vi "control_622x.vi"() -> ()   [LabVIEW 2018]
uses:
  <instrlib>/Keithley 622x LV 2009/Typedefs/KE622x -- On Off Control.ctl
  <instrlib>/Keithley 622x LV 2009/Keithley 622x.lvlib
panel:
  in  "Commande onglets":enum32{"Settings", "delta", "Hardware"}(tab)
  in  "start":bool
  in  "offset /A":dbl min=-0.1 max=0.1 format="%#.9g"
  in  "Source analog filter":bool
  in  "DMM range /V":dbl=1.0 min=0.01 max=100.0 format="%#.9g"
  in  "compliance /V":dbl=1.0 min=0.1 max=62.0 format="%#.9g"
  in  "AC frequency /Hz":dbl=17.0 min=1e-05 max=100000.0 format="%#.9g"
  in  "current /A (peak)":dbl=1e-09 min=-0.105 max=0.105 format="%#.9g"
  in  "Source autorange":bool
  in  "MODE":enum32{"source DC", "source AC ", "delta "}(radio)
  in  "source":bool
  in  "compliance abort":bool
  in  "DMM autorange":bool
  in  "exit":bool
  out "Graphe":dbl(graph)
  in  "VISA GPIB Resource":refnum<visa-resource-name>="GPIB0::4::INSTR"
  # "frequency TTL output at 0° on line 1\nfor Halbach, use the Trigger 1 connection to the Zurich instruments lock in"
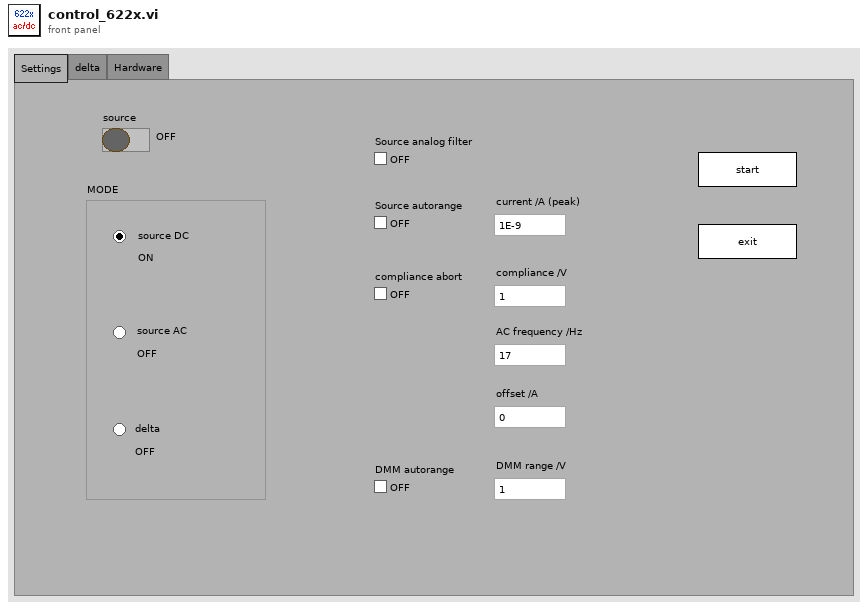
[diagram p1: front panel]
types:
  T1 = enum32{"invalid app kind", "Development System", "Run Time System", "Student Edition", "Embedded LabVIEW", "Evaluation", "Custom"}
  T2 = enum32{"Invalid", "Standard", "Closed", "Hidden", "Minimized", "Maximized"}
  T3 = typedef "Keithley 622x.lvlib/KE622x -- On Off Control.ctl" = enum16{"Off", "On"}
  T4 = cluster{"Core":cluster{"Current VI Reference":refnum<vi>, "Close Panel on Exit?":bool}, "VISA GPIB Resource":refnum<visa-resource-name>, "MODE":enum32{"source DC", "source AC ", "delta "}, "source ":bool, "Source analog filter":bool, "Source autorange ":bool, "compliance abort":bool, "DMM autorange":bool, "current /A (peak)":dbl, "compliance /V":dbl, "AC frequency /Hz":dbl, "DMM range /V ":dbl, "offset /A":dbl, "delta mode ON?":bool}
  T5 = cluster{"Current VI Reference":refnum<vi>, "Close Panel on Exit?":bool}
  T6 = typedef "Keithley 622x.lvlib/KE622x -- Current Range.ctl" = cluster{"Auto Range?":bool, "Man / Selected\nRange":T7}
  T7 = typedef "Keithley 622x.lvlib/KE622x -- Current Ranges.ctl" = enum16{"2nA", "20nA", "200nA", "2uA", "20uA", "200uA", "2mA", "20mA", "100mA"}
  T8 = cluster{"Source autorange ":bool, "Man / Selected\nRange":T7}
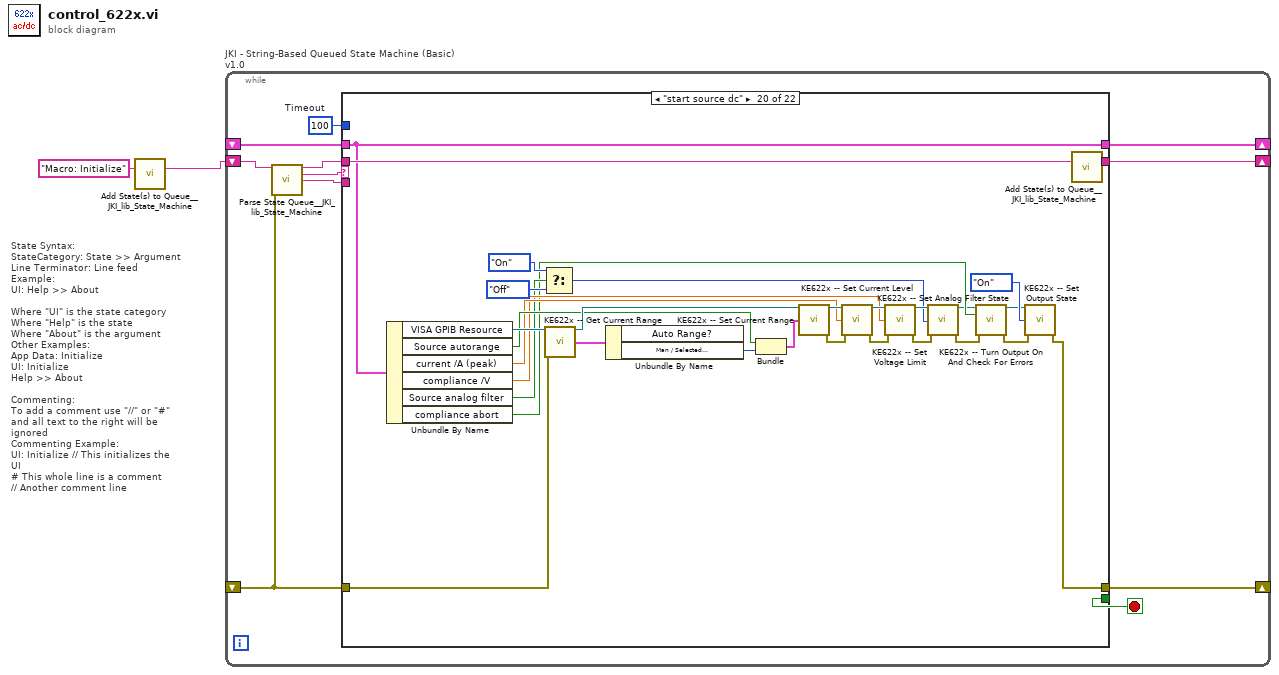
[diagram p0: block diagram]
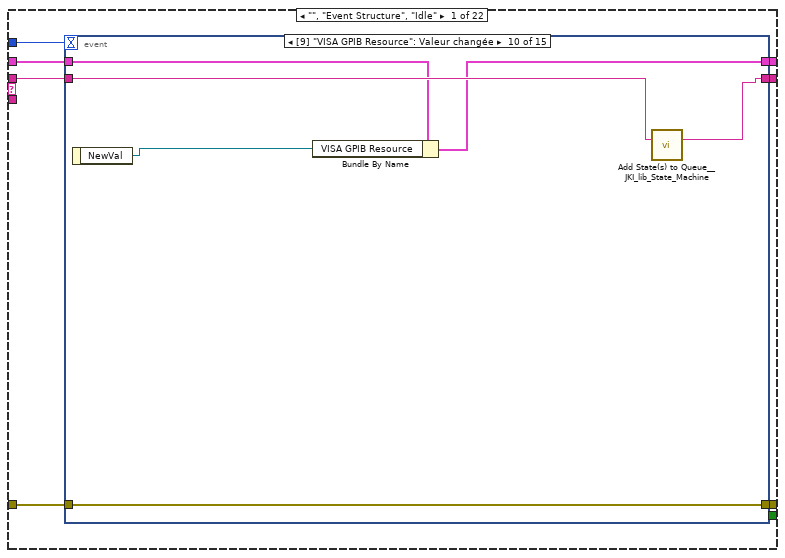
[diagram p2: hidden frame]
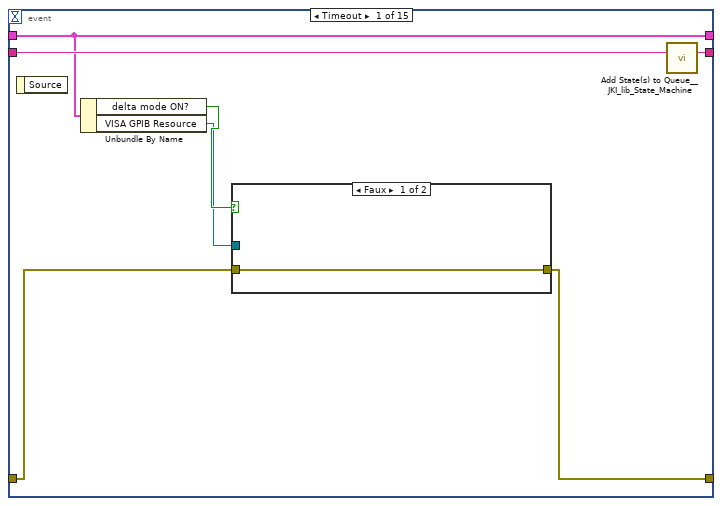
[diagram p3: hidden frame]
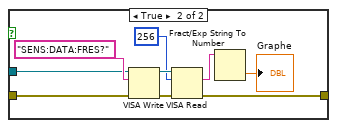
[diagram p4: hidden frame]
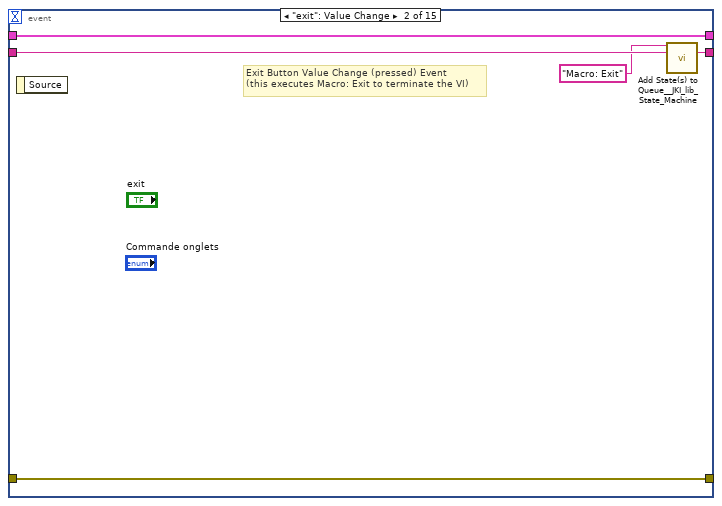
[diagram p5: hidden frame]
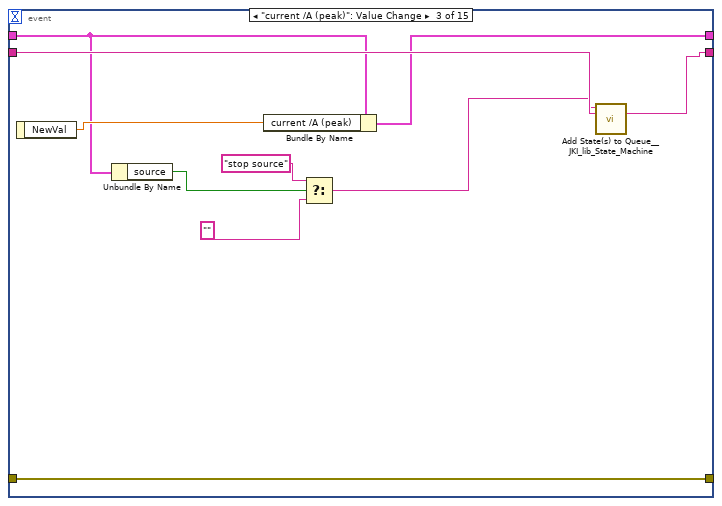
[diagram p6: hidden frame]
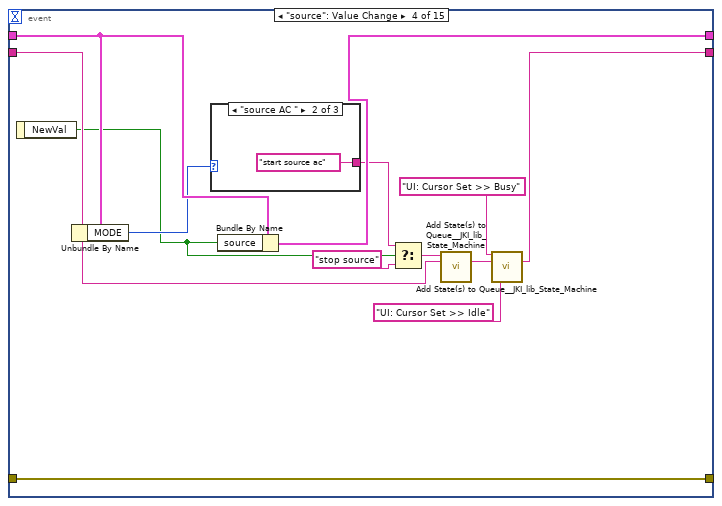
[diagram p7: hidden frame]
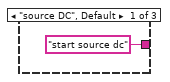
[diagram p8: hidden frame]
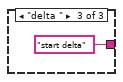
[diagram p9: hidden frame]
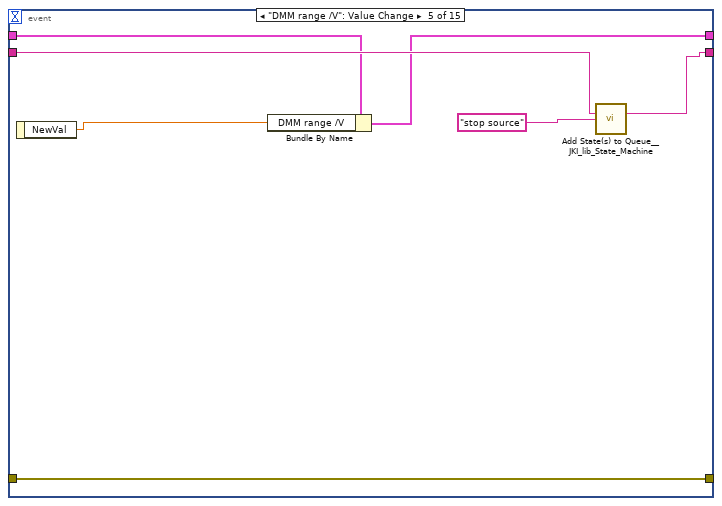
[diagram p10: hidden frame]
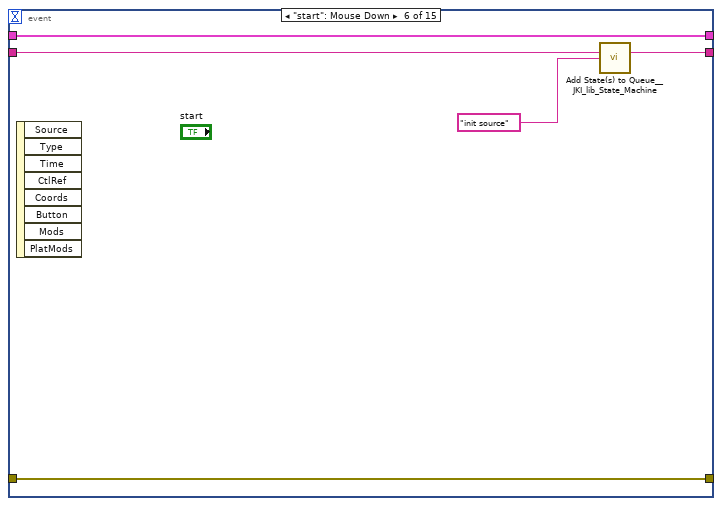
[diagram p11: hidden frame]
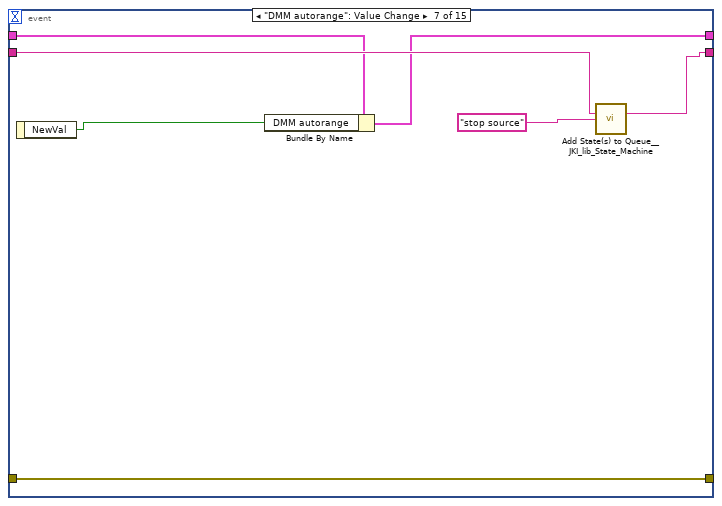
[diagram p12: hidden frame]
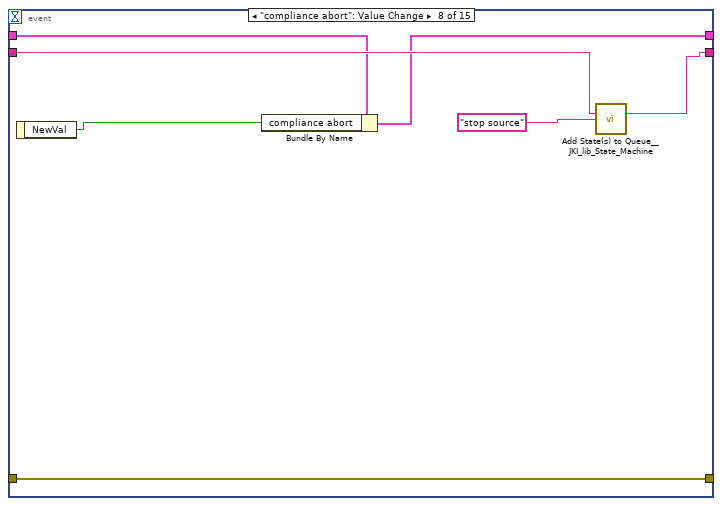
[diagram p13: hidden frame]
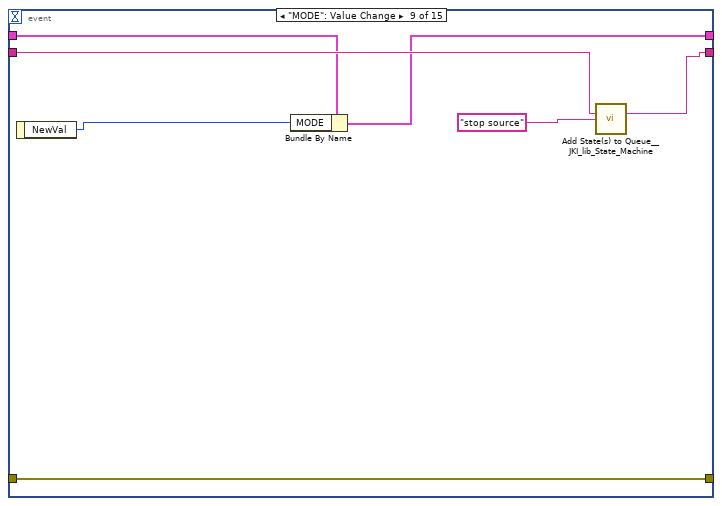
[diagram p14: hidden frame]
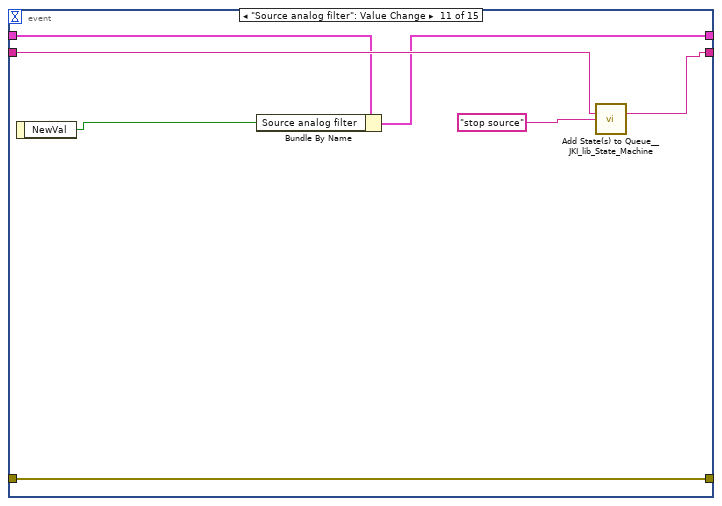
[diagram p15: hidden frame]
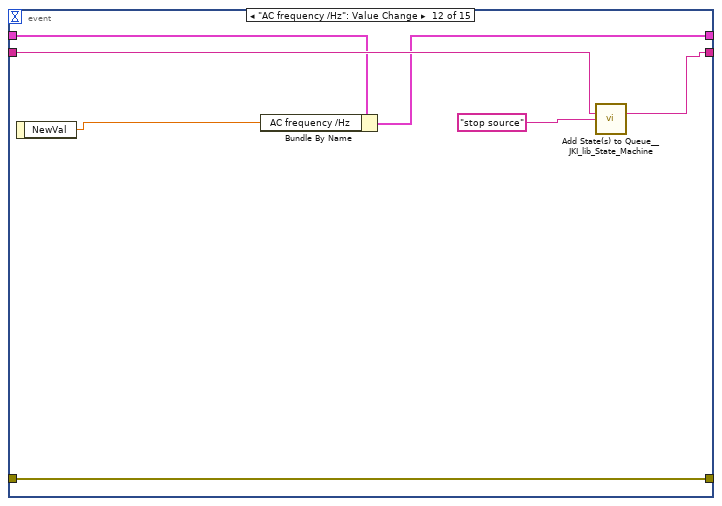
[diagram p16: hidden frame]
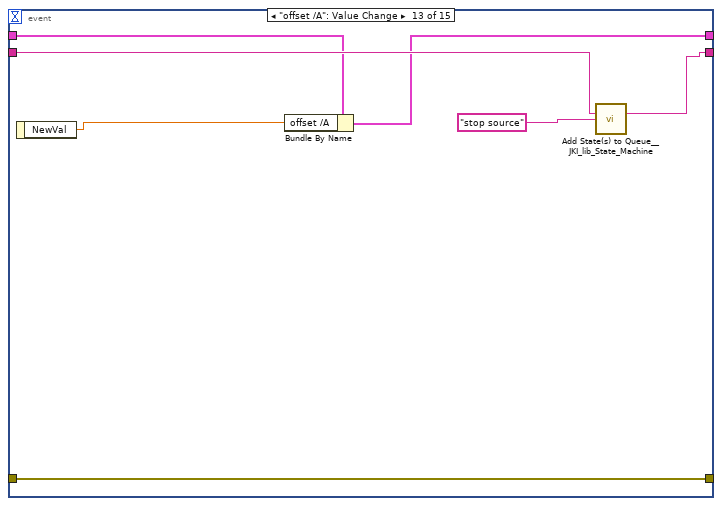
[diagram p17: hidden frame]
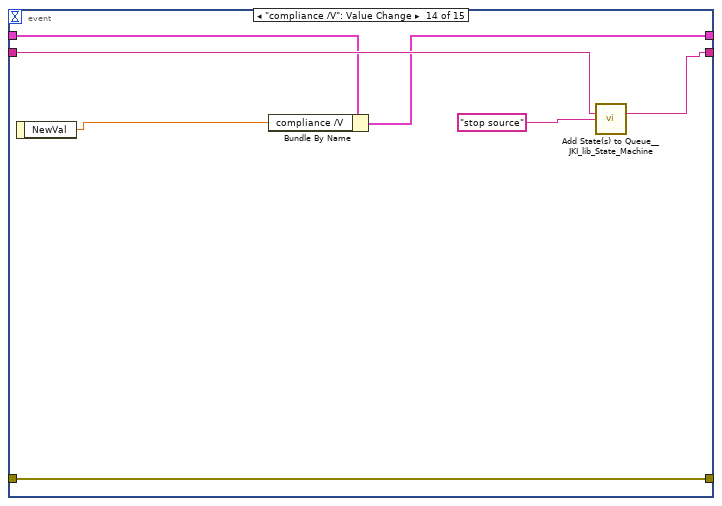
[diagram p18: hidden frame]
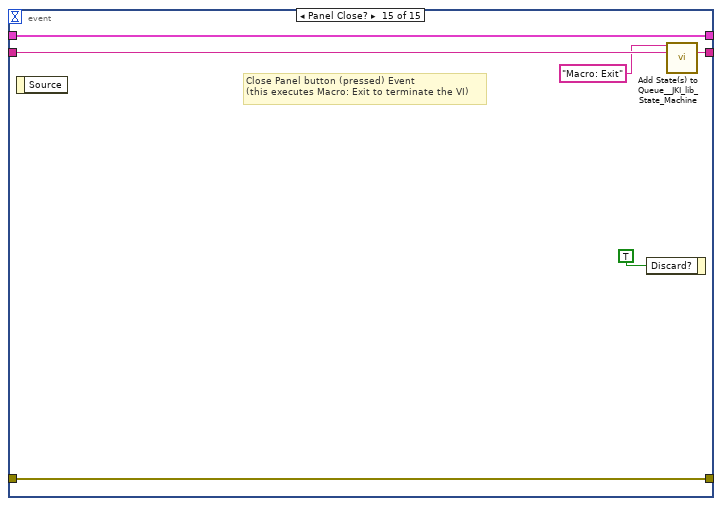
[diagram p19: hidden frame]
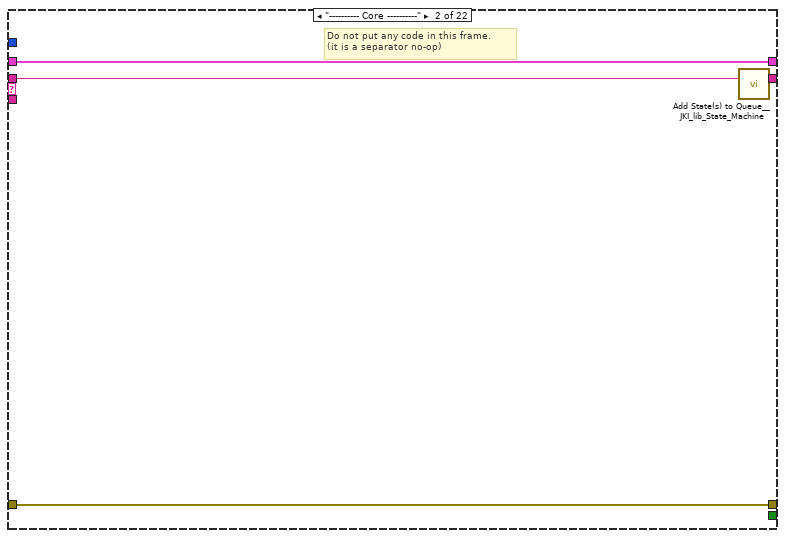
[diagram p20: hidden frame]
diagram:
  # "State Syntax:\nStateCategory: State >> Argument\nLine Terminator: Line feed\nExample:\nUI: Help >> About\n\nWhere \"UI\" is the state category\nWhere \"Help\" is the state\nWhere \"About\" is the argument\nOther Examples:\nApp Data: Initialize\nUI: Initialize\nHelp >> About\n\nCommenting:\nTo add a comment use \"//\" or \"#\" and all text to the right will be ignored\nCommenting Example:\nUI: Initialize // This initializes the UI\n# This whole line is a comment\n// Another comment line"
  n1 = call <vilib>:"Add State(s) to Queue__JKI_lib_State_Machine.vi"("State(s) in (\"\")"="Macro: Initialize") -> ("States Out"=w2:string)  [unwired: 14 in]
  n2 = while "JKI - String-Based Queued State Machine (Basic) v1.0" {
    shift-right: [w7] -> _
    shift-left: _ -> [w6]
    shift-right: [w3] -> _
    shift-left: _ -> [w4]
    shift-right: [w9] -> _
    shift-left: w2 -> [w10]
    stop <- w8 stop-if-true
    w5 = 100  # Timeout
    n3 = call <vilib>:"Parse State Queue__JKI_lib_State_Machine.vi"("State Queue"=w10, "Error In (no error)"=w4) -> ("Remaining States"=w12:string, "Current State"=w13:string, "Arguments"=w11:string)  [unwired: 11 in]
    n4 = case shown="\"start source dc\"" w13 {
      selector: w13 -> [_ _ w146 _ _ _ _ _ _ _ _ _ _ _ _ _ _ _ _ _ _ _]
      tunnel: w12 -> [w20 w145 w150 w168 w174 w179 w183 w201 w207 w211 w215 w221 w232 w258 w263 w274 w278 w291 w310 w339 w349 w362]
      tunnel: w11 -> [_ _ _ _ _ _ _ _ _ _ _ w216 w226 _ _ _ _ _ _ _ _ _]
      tunnel: w6 -> [w18 w142 w148 w159 w171 w177 w180 _ w202 w208 w213 w219 w228 w255 w260 w271 w275 w284 w308 w337 w347 w351]
      tunnel: [w17 w143 w152 w165 errorcluster {"status"=FALSE, "code"=0, "source"=""} ("error out") w176 w181 w184 w203 w209 w212 w217 w229 w256 w261 w272 w276 w280 w299 w311 w340 w355] -> w3
      tunnel: w4 -> [w16 w143 w151 w165 w170 w176 w181 w184 w204 w209 w212 w218 w230 w256 w261 w272 w276 w285 w301 w312 w341 w356]
      tunnel: [w19 w144 w149 w167 w173 w178 w182 w200 w206 w210 w214 w220 w231 w257 w262 w273 w277 w290 w309 w338 w348 w361] -> w9
      tunnel: [_ _ _ _ _ TRUE _ _ _ _ _ _ _ _ _ _ _ _ _ _ _ _] -> w8
      tunnel: [w15 w142 w148 w166 w171 w177 w180 w199 w202 w208 w213 w219 w228 w255 w260 w271 w275 w283 w308 w337 w347 w350] -> w7
      tunnel: w5 -> [w14 _ _ _ _ _ _ _ _ _ _ _ _ _ _ _ _ _ _ _ _ _]
      frame "", "Event Structure", "Idle" {
        n5 = event shown="[9] \"VISA GPIB Resource\": Valeur changée" {
          selector: _ -> [_ _ _ _ _ _ _ _ _ _ _ _ _ _ _]
          dyn-events: _ -> [_ _ _ _ _ _ _ _ _ _ _ _ _ _ _]
          timeout: w14 -> [_ _ _ _ _ _ _ _ _ _ _ _ _ _ _]
          tunnel: w20 -> [w27 w42 w51 w65 w73 w78 w85 w92 w99 w106 w112 w119 w126 w133 w141]
          tunnel: [w26 w41 w52 w57 w75 w80 w87 w94 w101 w107 w114 w121 w128 w135 w140] -> w19
          tunnel: w18 -> [w25 w39 w47 w62 w72 w76 w84 w91 w98 w105 w111 w118 w125 w132 w138]
          tunnel: [w21 w40 w48 w63 w69 w77 w81 w88 w95 w102 w108 w115 w122 w129 w139] -> w17
          tunnel: w16 -> [w22 w40 w48 w63 w69 w77 w81 w88 w95 w102 w108 w115 w122 w129 w139]
          tunnel: [w25 w39 w50 w64 w71 w76 w83 w90 w97 w104 w110 w117 w124 w131 w138] -> w15
          event Timeout {
            n6 = event-data() -> ()  [unwired: 1 in, 1 out]
            n7 = Unbundle By Name(w25) -> ("delta mode ON?"=w24:bool, "VISA GPIB Resource"=w23:refnum<visa-resource-name>)
            n8 = case shown="Faux" w24 {
              tunnel: w23 -> [_ w32]
              tunnel: w22 -> [w28 w31]
              tunnel: [w28 w30] -> w21
              frame False {
              }
              frame True {
                n9 = VISA Write(VISA resource name=w32, write buffer="SENS:DATA:FRES?" ("buffer d'écriture"), error in (no error)=w31) -> (VISA resource name out=w36:refnum<visa-resource-name>, error out=w35:errorcluster)  [unwired: 1 out]
                n10 = VISA Read(VISA resource name=w36, byte count=u32 256 ("nombre d'octets"), error in (no error)=w35) -> (read buffer=w33:string, error out=w30:errorcluster)  [unwired: 2 out]
                n11 = Fract/Exp String To Number(string=w33) -> (number=→"Graphe":dbl)  [unwired: 3 in, 1 out]
              }
            }
            n12 = call <vilib>:"Add State(s) to Queue__JKI_lib_State_Machine.vi"("State(s) in (\"\")"=w27) -> ("States Out"=w26:string)  [unwired: 14 in]
          }
          event "exit": Value Change {
            # "Exit Button Value Change (pressed) Event\n(this executes Macro: Exit to terminate the VI)"
            n13 = event-data() -> ()  [unwired: 1 in, 1 out]
            n14 = call <vilib>:"Add State(s) to Queue__JKI_lib_State_Machine.vi"("State(s) in Front (\"\")"="Macro: Exit", "State(s) in (\"\")"=w42) -> ("States Out"=w41:string)  [unwired: 13 in]
          }
          event "current /A (peak)": Value Change {
            n15 = event-data() -> ("NewVal"=w49:dbl)  [unwired: 1 in]
            n16 = Unbundle By Name(w47) -> ("source"=w46:bool)
            n17 = Bundle By Name(cluster=w47, "current /A (peak)"=w49) -> (w50:T4)
            n18 = Select(t="stop source", s=w46, f="") -> (s? t:f=w43:string)
            n19 = call <vilib>:"Add State(s) to Queue__JKI_lib_State_Machine.vi"("State(s) in Front (\"\")"=w43, "State(s) in (\"\")"=w51) -> ("States Out"=w52:string)  [unwired: 13 in]
          }
          event "source": Value Change {
            n20 = event-data() -> ("NewVal"=w53:bool)  [unwired: 1 in]
            n21 = Unbundle By Name(w62) -> ("MODE"=w59:enum32{"source DC", "source AC ", "delta "})
            n22 = case shown="\"source AC \"" w59 {
              tunnel: ["start source dc" "start source ac" "start delta"] -> w58
              frame "source DC", Default {
              }
              frame "source AC " {
              }
              frame "delta " {
              }
            }
            n23 = Bundle By Name(cluster=w62, "source"=w53) -> (w64:T4)
            n24 = Select(t=w58, s=w53, f="stop source") -> (s? t:f=w61:string)
            n25 = call <vilib>:"Add State(s) to Queue__JKI_lib_State_Machine.vi"("State(s) in Front (\"\")"=w61, "State(s) in (\"\")"=w65) -> ("States Out"=w56:string)  [unwired: 13 in]
            n26 = call <vilib>:"Add State(s) to Queue__JKI_lib_State_Machine.vi"("State(s) in Front (\"\")"="UI: Cursor Set >> Busy", "State(s) in (\"\")"=w56, "State(s) at Back (\"\")"="UI: Cursor Set >> Idle") -> ("States Out"=w57:string)  [unwired: 12 in]
          }
          event "DMM range /V": Value Change {
            n27 = event-data() -> ("NewVal"=w70:dbl)  [unwired: 1 in]
            n28 = Bundle By Name(cluster=w72, "DMM range /V"=w70) -> (w71:T4)
            n29 = call <vilib>:"Add State(s) to Queue__JKI_lib_State_Machine.vi"("State(s) in (\"\")"=w73, "State(s) at Back (\"\")"="stop source") -> ("States Out"=w75:string)  [unwired: 13 in]
          }
          event "start": Mouse Down {
            n30 = event-data() -> ()  [unwired: 1 in, 8 out]
            n31 = call <vilib>:"Add State(s) to Queue__JKI_lib_State_Machine.vi"("State(s) in (\"\")"=w78, "State(s) at Back (\"\")"="init source") -> ("States Out"=w80:string)  [unwired: 13 in]
          }
          event "DMM autorange": Value Change {
            n32 = event-data() -> ("NewVal"=w82:bool)  [unwired: 1 in]
            n33 = Bundle By Name(cluster=w84, "DMM autorange"=w82) -> (w83:T4)
            n34 = call <vilib>:"Add State(s) to Queue__JKI_lib_State_Machine.vi"("State(s) in (\"\")"=w85, "State(s) at Back (\"\")"="stop source") -> ("States Out"=w87:string)  [unwired: 13 in]
          }
          event "compliance abort": Value Change {
            n35 = event-data() -> ("NewVal"=w89:bool)  [unwired: 1 in]
            n36 = Bundle By Name(cluster=w91, "compliance abort"=w89) -> (w90:T4)
            n37 = call <vilib>:"Add State(s) to Queue__JKI_lib_State_Machine.vi"("State(s) in (\"\")"=w92, "State(s) at Back (\"\")"="stop source") -> ("States Out"=w94:string)  [unwired: 13 in]
          }
          event "MODE": Value Change {
            n38 = event-data() -> ("NewVal"=w96:enum32{"source DC", "source AC ", "delta "})  [unwired: 1 in]
            n39 = Bundle By Name(cluster=w98, "MODE"=w96) -> (w97:T4)
            n40 = call <vilib>:"Add State(s) to Queue__JKI_lib_State_Machine.vi"("State(s) in (\"\")"=w99, "State(s) at Back (\"\")"="stop source") -> ("States Out"=w101:string)  [unwired: 13 in]
          }
          event "VISA GPIB Resource": Value Change {
            n41 = event-data() -> ("NewVal"=w103:refnum<visa-resource-name>)  [unwired: 1 in]
            n42 = Bundle By Name(cluster=w105, "VISA GPIB Resource"=w103) -> (w104:T4)
            n43 = call <vilib>:"Add State(s) to Queue__JKI_lib_State_Machine.vi"("State(s) in (\"\")"=w106) -> ("States Out"=w107:string)  [unwired: 14 in]
          }
          event "Source analog filter": Value Change {
            n44 = event-data() -> ("NewVal"=w109:bool)  [unwired: 1 in]
            n45 = Bundle By Name(cluster=w111, "Source analog filter"=w109) -> (w110:T4)
            n46 = call <vilib>:"Add State(s) to Queue__JKI_lib_State_Machine.vi"("State(s) in (\"\")"=w112, "State(s) at Back (\"\")"="stop source") -> ("States Out"=w114:string)  [unwired: 13 in]
          }
          event "AC frequency /Hz": Value Change {
            n47 = event-data() -> ("NewVal"=w116:dbl)  [unwired: 1 in]
            n48 = Bundle By Name(cluster=w118, "AC frequency /Hz"=w116) -> (w117:T4)
            n49 = call <vilib>:"Add State(s) to Queue__JKI_lib_State_Machine.vi"("State(s) in (\"\")"=w119, "State(s) at Back (\"\")"="stop source") -> ("States Out"=w121:string)  [unwired: 13 in]
          }
          event "offset /A": Value Change {
            n50 = event-data() -> ("NewVal"=w123:dbl)  [unwired: 1 in]
            n51 = Bundle By Name(cluster=w125, "offset /A"=w123) -> (w124:T4)
            n52 = call <vilib>:"Add State(s) to Queue__JKI_lib_State_Machine.vi"("State(s) in (\"\")"=w126, "State(s) at Back (\"\")"="stop source") -> ("States Out"=w128:string)  [unwired: 13 in]
          }
          event "compliance /V": Value Change {
            n53 = event-data() -> ("NewVal"=w130:dbl)  [unwired: 1 in]
            n54 = Bundle By Name(cluster=w132, "compliance /V"=w130) -> (w131:T4)
            n55 = call <vilib>:"Add State(s) to Queue__JKI_lib_State_Machine.vi"("State(s) in (\"\")"=w133, "State(s) at Back (\"\")"="stop source") -> ("States Out"=w135:string)  [unwired: 13 in]
          }
          event Panel Close? {
            # "Close Panel button (pressed) Event\n(this executes Macro: Exit to terminate the VI)"
            n56 = event-data() -> ()  [unwired: 1 in, 1 out]
            n57 = event-data("Discard?"=TRUE) -> ()  [unwired: 1 in, 1 out]
            n58 = call <vilib>:"Add State(s) to Queue__JKI_lib_State_Machine.vi"("State(s) in Front (\"\")"="Macro: Exit", "State(s) in (\"\")"=w141) -> ("States Out"=w140:string)  [unwired: 13 in]
          }
        }
      }
      frame "---------- Core ----------" {
        # "Do not put any code in this frame.\n(it is a separator no-op)"
        n59 = call <vilib>:"Add State(s) to Queue__JKI_lib_State_Machine.vi"("State(s) in (\"\")"=w145) -> ("States Out"=w144:string)  [unwired: 14 in]
      }
      frame Default {
        w155 = 42 items=["No error", "Argument error", "Memory is full", "Out of zone", "End of file", "File already open", "Generic file I/O error", "File not found", "File permission error", "Disk is full", "Duplicate path", "Too many files open", "System feature not enabled", "Resource file not found", "Cannot add resource", "Resource not found", "Image not found", "Image memory error", "Pen does not exist", "Config type invalid", "Config token not found", "Config parse error", "Config memory error", "Bad external code format", "Bad external code offset", "External code not present", "Null window", "Destroy window error", "Null menu", "Print aborted", "Bad print record", "Print driver error", "Windows error during printing", "Memory error during printing", "Print dialog error", "Generic print error", "Invalid device refnum", "Device not found", "Device parameter error", "Device unit error", "Cannot open device", "Device call aborted", "Generic error", "Cancelled by user", "Object ID too low", "Object ID too high", "Object not in heap", "Unknown heap", "Unknown object (invalid DefProc)", "Unknown object (DefProc not in table)", "Message out of range", "Invalid (null) method", "Unknown message", "Manager call not supported", "Bad address", "Network operation in progress", "Network operation timed out", "Connection is busy", "Network attribute not supported", "Network error", "Address in use", "System out of memory", "Connection aborted", "Connection refused", "Not connected", "Already connected", "Connection closed", "Initialization error (interapplication manager)", "Bad occurrence", "Wait on unbound occurrence handler", "Occurrence queue overflow", "Datalog type conflict", "Unused", "Unrecognized type (interapplication manager)", "Memory corrupt", "Failed to make temporary DLL", "Old CIN version", "Drag socket not found", "Failed to load drop-object", "Failed to register OLE object", "Failed to release OLE object", "Format specifier type mismatch", "Unknown format specifier", "Too few format specifiers", "Too many format specifiers", "Scan failed", "Newer CIN version", "Error converting to variant", "Runtime menu error", "Password tampered", "Variant attribute not found", "Incompatible variant data type", "Event data is not available", "Event Store is not present", "Occurrence is not found", "Event Queue is not created", "Event info is not available", "Refnum passed is NULL", "Error retrieving Class GUID", "Error retrieving CoClass GUID", "Error retrieving TypeLib GUID.", "Bad built application magic bytes.", "Specific driver is different from the specific driver associated with the Logical Name.", "There is no session opened to the class driver.", "Max Error", "MAX - Error with config objects", "MAX - Error loading configuration", "MAX - Group not supported"]
        # "Current State"
        # "Do not delete, rename, or modify this frame.\n(this is used to capture unhandled states and typos)"
        # "Handle mistyped state name (developer tool)"
        n60 = Format Into String(format string="Software Exception: Unhandled State \"%s\"." ("message"), error in=w151, w146) -> (resulting string=w154:string, error out=w153:errorcluster)  [unwired: 1 in]
        n61 = call <vilib>:"Error Cluster From Error Code.vi"("show call chain? (False)"=TRUE, "error in (no error)"=w153, "error message (\"\")"=w154, "error code (0)"=w155) -> ("error out"=w152:errorcluster)  [unwired: 5 in]
        n62 = call <vilib>:"Add State(s) to Queue__JKI_lib_State_Machine.vi"("State(s) in (\"\")"=w150) -> ("States Out"=w149:string)  [unwired: 14 in]
      }
      frame "Initialize Core Data" {
        # "Do not delete, rename, or modify this frame.\n(this is used to determine panel behavior on exit)"
        # "originally closed?"
        # "exe?"
        # "If panel starts closed or is an EXE, then close it when we exit"
        n63 = property class="VI"() -> ("Front Panel.Open"=w164:bool)  [unwired: 2 in, 2 out]
        n64 = property class="App"() -> ("App.Kind"=w163:T1)  [unwired: 2 in, 2 out]
        n65 = control-ref of="Current VI Reference"() -> (w157:refnum<vi>)
        n66 = Not(x=w164) -> (.not. x?=w161:bool)
        n67 = Equal?(x=w163, y=T1."Run Time System" ("Application:Kind")) -> (x = y?=w160:bool)
        n68 = Or(x=w161, y=w160) -> (x .or. y?=w158:bool)
        n69 = Bundle By Name(cluster=w159, "Core.Current VI Reference"=w157, "Core.Close Panel on Exit?"=w158) -> (w166:T4)
        n70 = call <vilib>:"Add State(s) to Queue__JKI_lib_State_Machine.vi"("State(s) in (\"\")"=w168) -> ("States Out"=w167:string)  [unwired: 14 in]
      }
      frame "Error Handler" {
        # "Unhandled Error -- Display it"
        # "Handle any errors here.\nYou can also output any states to clean-up after errors occur"
        # "Clear error"
        n71 = call <vilib>:"General Error Handler.vi"("error in (no error)"=w170) -> ()  [unwired: 10 in, 5 out]
        n72 = call <vilib>:"Add State(s) to Queue__JKI_lib_State_Machine.vi"("State(s) in Front (\"\")"="/* Post Error States", "State(s) in (\"\")"=w174) -> ("States Out"=w173:string)  [unwired: 13 in]
      }
      frame "Exit" {
        # "Do not put any code in this frame.\n(No errors that occur here will be handled.)"
        n73 = call <vilib>:"Add State(s) to Queue__JKI_lib_State_Machine.vi"("State(s) in (\"\")"=w179) -> ("States Out"=w178:string)  [unwired: 14 in]
      }
      frame "---------- Data ----------" {
        # "Do not put any code in this frame.\n(It is a separator no-op. You can make a copy of this frame to create a new Data frame)"
        n74 = call <vilib>:"Add State(s) to Queue__JKI_lib_State_Machine.vi"("State(s) in (\"\")"=w183) -> ("States Out"=w182:string)  [unwired: 14 in]
      }
      frame "Data: Initialize" {
        w185 = FALSE  # delta mode ON?
        w198 = T5 {"Current VI Reference"=refnum, "Close Panel on Exit?"=FALSE}  # Core
        # "Initialize the shift-register data, here.\n(data names are defined by what you wire into the bundle function)"
        n75 = Bundle("Core"=w198, "VISA GPIB Resource"="VISA GPIB Resource", "MODE"="MODE", "source"="source", "Source analog filter"="Source analog filter", "Source autorange"="Source autorange", "compliance abort"="compliance abort", "DMM autorange"="DMM autorange", "current /A (peak)"="current /A (peak)", "compliance /V"="compliance /V", "AC frequency /Hz"="AC frequency /Hz", "DMM range /V"="DMM range /V", "offset /A"="offset /A", "delta mode ON?"=w185) -> (w199:T4)  [unwired: 1 in]
        n76 = call <vilib>:"Add State(s) to Queue__JKI_lib_State_Machine.vi"("State(s) in (\"\")"=w201) -> ("States Out"=w200:string)  [unwired: 14 in]
      }
      frame "Data: Cleanup" {
        # "Cleanup any data and references, here.\n(this is called automatically, by the Macro: Exit)"
        n77 = Unbundle By Name(w202) -> ("Core.Current VI Reference"=w205:refnum<vi>)
        n78 = Close Reference(reference=w205, error in (no error)=w204) -> (error out=w203:errorcluster)
        n79 = call <vilib>:"Add State(s) to Queue__JKI_lib_State_Machine.vi"("State(s) in (\"\")"=w207) -> ("States Out"=w206:string)  [unwired: 14 in]
      }
      frame "---------- UI ----------" {
        # "Do not put any code in this frame.\n(It is a separator no-op. You can make a copy of this frame to create a new UI frame)"
        n80 = call <vilib>:"Add State(s) to Queue__JKI_lib_State_Machine.vi"("State(s) in (\"\")"=w211) -> ("States Out"=w210:string)  [unwired: 14 in]
      }
      frame "UI: Initialize" {
        # "Initialize the User Interface, here.\n(this is called automatically, by the Macro: Init)"
        n81 = call <vilib>:"Add State(s) to Queue__JKI_lib_State_Machine.vi"("State(s) in (\"\")"=w215) -> ("States Out"=w214:string)  [unwired: 14 in]
      }
      frame "UI: Cursor Set" {
        # "Argument"
        # "Set and Unset Cursor Busy.\n(Usage: \"UI: Cursor Set >> Busy|Idle\")"
        n82 = case shown="\"Idle\", Par défaut" w216 {
          tunnel: w218 -> [w223 w225]
          tunnel: [w222 w224] -> w217
          frame "Idle", Default {
            n83 = call <vilib>:"Unset Busy.vi"("error in (no error)"=w223) -> ("error out"=w222:errorcluster)  [unwired: 10 in]
          }
          frame "Busy" {
            n84 = call <vilib>:"Set Busy.vi"("error in (no error)"=w225) -> ("error out"=w224:errorcluster)  [unwired: 9 in, 1 out]
          }
        }
        n85 = call <vilib>:"Add State(s) to Queue__JKI_lib_State_Machine.vi"("State(s) in (\"\")"=w221) -> ("States Out"=w220:string)  [unwired: 14 in]
      }
      frame "UI: Front Panel State" {
        # "Argument"
        # "Set Front Panel Open or Closed\n(Usage: \"UI: Front Panel State >> Open|Close\")"
        n86 = Unbundle By Name(w228) -> ("Core.Current VI Reference"=w227:refnum<vi>)
        n87 = case shown="\"Open\", Par défaut" w226 {
          tunnel: w230 -> [w236 w249]
          tunnel: [w238 w250] -> w229
          tunnel: w227 -> [w237 w247]
          frame "Open", Default {
            n88 = property class="VI"(reference=w237, error in=w236) -> (reference out=w234:refnum<vi>, error out=w235:errorcluster, "Front Panel.Open"=w233:bool)
            n89 = case shown="Vrai" w233 {
              tunnel: [w241 w244] -> w238
              tunnel: w235 -> [w240 w244]
              tunnel: w234 -> [w239 _]
              frame False {
                n90 = invoke class="VI" method="FA.Ouvrir"(reference=w239, error in=w240, "Activate"=TRUE, "State"=T2."Standard") -> (error out=w241:errorcluster)  [unwired: 1 in, 4 out]
              }
              frame True {
              }
            }
          }
          frame "Close" {
            n91 = property class="VI"(reference=w247, error in=w249) -> (reference out=w246:refnum<vi>, error out=w248:errorcluster, "Front Panel.Open"=w245:bool)
            n92 = case shown="Vrai" w245 {
              tunnel: [w251 w254] -> w250
              tunnel: w248 -> [w251 w253]
              tunnel: w246 -> [_ w252]
              frame False {
              }
              frame True {
                n93 = invoke class="VI" method="FA.Fermer"(reference=w252, error in=w253) -> (error out=w254:errorcluster)  [unwired: 1 in, 2 out]
              }
            }
          }
        }
        n94 = call <vilib>:"Add State(s) to Queue__JKI_lib_State_Machine.vi"("State(s) in (\"\")"=w232) -> ("States Out"=w231:string)  [unwired: 14 in]
      }
      frame "---------- Macro ----------" {
        # "Do not put any code in this frame.\n(It is a separator no-op. You can make a copy of this frame to create a new Macro frame)"
        n95 = call <vilib>:"Add State(s) to Queue__JKI_lib_State_Machine.vi"("State(s) in (\"\")"=w258) -> ("States Out"=w257:string)  [unwired: 14 in]
      }
      frame "Macro: Initialize" {
        # "Initialization Macro\n(This is called once, when the VI starts)"
        n96 = call <vilib>:"Add State(s) to Queue__JKI_lib_State_Machine.vi"("State(s) in Front (\"\")"="UI: Cursor Set >> Busy\nData: Initialize\nInitialize Core Data\nUI: Initialize\nUI: Front Panel State >> Open\nUI: Cursor Set >> Idle", "State(s) in (\"\")"=w263) -> ("States Out"=w262:string)  [unwired: 13 in]
      }
      frame "Macro: Exit" {
        # "Exit Macro\n(This is called once, when the VI exits)"
        n97 = Unbundle By Name(w271) -> ("Core.Close Panel on Exit?"=w270:bool)
        n98 = Select(t="UI: Front Panel State >> Close", s=w270, f="") -> (s? t:f=w267:string)
        n99 = call <vilib>:"Add State(s) to Queue__JKI_lib_State_Machine.vi"("State(s) in Front (\"\")"="stop source" ("State(s) in Front (\"\")"), "State(s) in (\"\")"=w267, "State(s) at Back (\"\")"="Data: Cleanup\nExit") -> ("States Out"=w265:string)  [unwired: 12 in]
        n100 = call <vilib>:"Add State(s) to Queue__JKI_lib_State_Machine.vi"("State(s) in Front (\"\")"=w265, "State(s) in (\"\")"=w274) -> ("States Out"=w273:string)  [unwired: 13 in]
      }
      frame "---------- my state machine ----------" {
        # "Template Separator\n(You can make a copy of, or modify, this frame)"
        n101 = call <vilib>:"Add State(s) to Queue__JKI_lib_State_Machine.vi"("State(s) in (\"\")"=w278) -> ("States Out"=w277:string)  [unwired: 14 in]
      }
      frame "stop source" {
        # "clear error if the source is not active"
        n102 = Unbundle By Name(w284) -> ("VISA GPIB Resource"=w289:refnum<visa-resource-name>)
        n103 = call <instrlib>:"KE622x -- Get Output State.vi"("Resource In"=w289, "error in (no error)"=w285) -> ("Resource Out (dupl)"=w287:refnum<visa-resource-name>, "Output State"=w288:T3, "error out"=w286:errorcluster)  [unwired: 11 in]
        n104 = case shown="\"Off\", Par défaut" w288 {
          tunnel: w287 -> [_ w297]
          tunnel: w286 -> [w292 w296]
          tunnel: [w292 w293] -> w281
          frame "Off", Default {
          }
          frame "On" {
            n105 = call <instrlib>:"KE622x -- Set Output State.vi"("Resource In"=w297, "Output State"=KE622x_--_On_Off_Control."Off", "error in (no error)"=w296) -> ("error out"=w294:errorcluster)  [unwired: 11 in, 1 out]
            n106 = property on="source" class="Bool (strict)"(error in=w294, "Value"=FALSE ("source on")) -> (error out=w293:errorcluster)  [unwired: 1 in, 1 out]
          }
        }
        n107 = Bundle By Name(cluster=w284, "delta mode ON?"=FALSE) -> (w283:T4)
        n108 = call <vilib>:"Clear Errors.vi"("error in (no error)"=w281, "specific error code to clear (0: all)"=0) -> ("error out"=w280:errorcluster)  [unwired: 4 in, 1 out]
        n109 = call <vilib>:"Add State(s) to Queue__JKI_lib_State_Machine.vi"("State(s) in (\"\")"=w291) -> ("States Out"=w290:string)  [unwired: 14 in]
      }
      frame "init source" {
        n110 = Unbundle By Name(w308) -> ("VISA GPIB Resource"=w300:refnum<visa-resource-name>)
        n111 = VISA Write(VISA resource name=w300, write buffer=":sour:wave:abor\n:outp:stat off\n*rst" ("buffer à écrire"), error in (no error)=w301) -> (VISA resource name out=w302:refnum<visa-resource-name>, error out=w304:errorcluster)  [unwired: 1 out]
        n112 = call "wait"("error in (no error)"=w304, "Delay Time (s)"=1.0) -> ("error out"=w303:errorcluster)  [unwired: 9 out]
        n113 = VISA Write(VISA resource name=w302, write buffer=":outp:ish olow\n:outp:lte off" ("buffer à écrire"), error in (no error)=w303) -> (error out=w299:errorcluster)  [unwired: 2 out]
        n114 = call <vilib>:"Add State(s) to Queue__JKI_lib_State_Machine.vi"("State(s) in (\"\")"=w310) -> ("States Out"=w309:string)  [unwired: 14 in]
      }
      frame "start source dc" {
        n115 = Unbundle By Name(w337) -> ("VISA GPIB Resource"=w333:refnum<visa-resource-name>, "Source autorange"=w329:bool, "current /A (peak)"=w327:dbl, "compliance /V"=w326:dbl, "Source analog filter"=w323:bool, "compliance abort"=w318:bool)
        n116 = Select(t=KE622x_--_On_Off_Control."On" ("Analog Filter State"), s=w323, f=KE622x_--_On_Off_Control."Off" ("Analog Filter State")) -> (s? t:f=w322:T3)
        n117 = call <instrlib>:"KE622x -- Get Current Range.vi"("Resource In"=w333, "error in (no error)"=w312) -> ("Resource Out (dupl)"=w332:refnum<visa-resource-name>, "Current Range"=w331:T6)  [unwired: 11 in, 1 out]
        n118 = Unbundle By Name(w331) -> ("Man / Selected\nRange"=w330:T7)  [unwired: 1 out]
        n119 = Bundle("Source autorange"=w329, "Man / Selected\nRange"=w330) -> (w328:T8)  [unwired: 1 in]
        n120 = call <instrlib>:"KE622x -- Set Current Range.vi"("Resource In"=w332, "Current Range In"=w328) -> ("Resource Out (dupl)"=w336:refnum<visa-resource-name>, "error out"=w320:errorcluster)  [unwired: 11 in, 1 out]
        n121 = call <instrlib>:"KE622x -- Set Current Level.vi"("Resource In"=w336, "Current Level (A) In"=w327, "error in (no error)"=w320) -> ("Resource Out (dupl)"=w335:refnum<visa-resource-name>, "error out"=w319:errorcluster)  [unwired: 10 in, 1 out]
        n122 = call <instrlib>:"KE622x -- Set Voltage Limit.vi"("Resource In"=w335, "Voltage Limit (V)"=w326, "error in (no error)"=w319) -> ("Resource Out (dupl)"=w334:refnum<visa-resource-name>, "error out"=w315:errorcluster)  [unwired: 11 in]
        n123 = call <instrlib>:"KE622x -- Set Analog Filter State.vi"("Resource In"=w334, "Analog Filter State"=w322, "error in (no error)"=w315) -> ("Resource Out (dupl)"=w317:refnum<visa-resource-name>, "error out"=w314:errorcluster)  [unwired: 11 in]
        n124 = call <instrlib>:"KE622x -- Turn Output On And Check For Errors.vi"("Resource In"=w317, "Turn Off Output If Compliance?"=w318, "error in (no error)"=w314) -> ("Resource Out (dupl)"=w316:refnum<visa-resource-name>, "error out"=w313:errorcluster)  [unwired: 9 in, 2 out]
        n125 = call <instrlib>:"KE622x -- Set Output State.vi"("Resource In"=w316, "Output State"=KE622x_--_On_Off_Control."On", "error in (no error)"=w313) -> ("error out"=w311:errorcluster)  [unwired: 11 in, 1 out]
        n126 = call <vilib>:"Add State(s) to Queue__JKI_lib_State_Machine.vi"("State(s) in (\"\")"=w339) -> ("States Out"=w338:string)  [unwired: 14 in]
      }
      frame "start source ac" {
        n127 = Unbundle By Name(w347) -> ("VISA GPIB Resource"=w346:refnum<visa-resource-name>, "current /A (peak)"=w344:dbl, "compliance /V"=w343:dbl, "AC frequency /Hz"=w342:dbl, "offset /A"=w345:dbl)  [unwired: 2 out]
        n128 = call "SIN_KE622x_.vi"("frequency /HZ"=w342, "compliance /V"=w343, "entrée d'erreur (pas d'erreur)"=w341, "amplitude /A"=w344, "offset /A"=w345, "VISA GPIB Resource"=w346) -> ("error out"=w340:errorcluster)  [unwired: 1 out]
        n129 = call <vilib>:"Add State(s) to Queue__JKI_lib_State_Machine.vi"("State(s) in (\"\")"=w349) -> ("States Out"=w348:string)  [unwired: 14 in]
      }
      frame "start delta" {
        n130 = Unbundle By Name(w351) -> ("VISA GPIB Resource"=w360:refnum<visa-resource-name>, "compliance abort"=w359:bool, "DMM autorange"=w358:bool, "current /A (peak)"=w357:dbl, "compliance /V"=w353:dbl, "DMM range /V"=w354:dbl)
        n131 = call "ke622x_2182a_setdelta.vi"("622x VISA"=w360, "range /V"=w354, "compliance abort"=w359, "DMM auto range"=w358, "current /A"=w357, "error in (no error)"=w356, "compliance /V"=w353) -> ("error out"=w355:errorcluster)  [unwired: 7 in, 1 out]
        n132 = Bundle By Name(cluster=w351, "delta mode ON?"=TRUE) -> (w350:T4)
        n133 = call <vilib>:"Add State(s) to Queue__JKI_lib_State_Machine.vi"("State(s) in (\"\")"=w362) -> ("States Out"=w361:string)  [unwired: 14 in]
      }
    }
  }
